vi "capacitance navigation v2.vi"() -> ()   [LabVIEW 2021]
uses:
  <userlib>/Nanonis Prog Interface V5/Nanonis Prog Interface.lvlib
panel:
  out "Delta reached?":bool
  out "Cap reached?":bool
  in  "Cap threshold (pA)":dbl=500.0
  in  "Stop when \nthreshold reached":bool=TRUE
  in  "Stop when delta \nthreshold reached":bool=TRUE
  in  "Delta cap threshold (pA)":dbl=1.0
  in  "pause":bool
  in  "Delete First Entry":bool
  in  "Time between averages (ms)":u32
  out "Avg index":i32
  in  "Averages":i32=50
  in  "milliseconds to wait":u32=1000
  in  "stop":bool
  in  "?":bool
  in  "Max Steps":u16=500
  in  "Direction":enum16{"X +", "X -", "Y +", "Y -", "Z +", "Z -"}(ring)
  out "Delta":cluster{"index":i32, sgl}[](graph)
  in  "Number of Steps":u16=50
  out "Capacitance":cluster{"index":i32, sgl}[](graph)
  in  "Frequency (Hz)":sgl=261.0
  in  "Amplitude (V)":sgl=260.0
  # "Max Steps On"
  # "Max Steps Off"
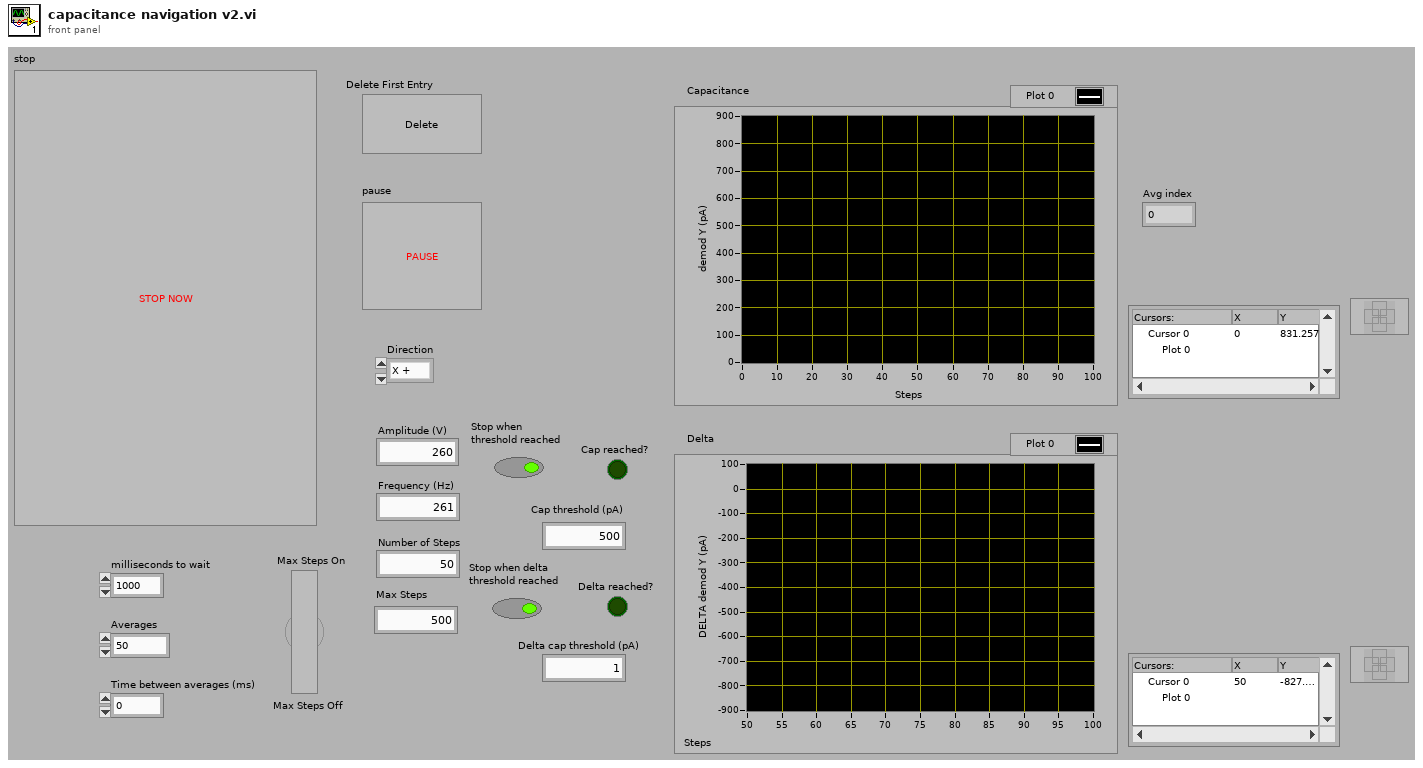
[diagram p1: front panel]
types:
  T1 = enum8{"Group 1", "Group 2", "Group 3", "Group 4", "Group 5", "Group 6"}
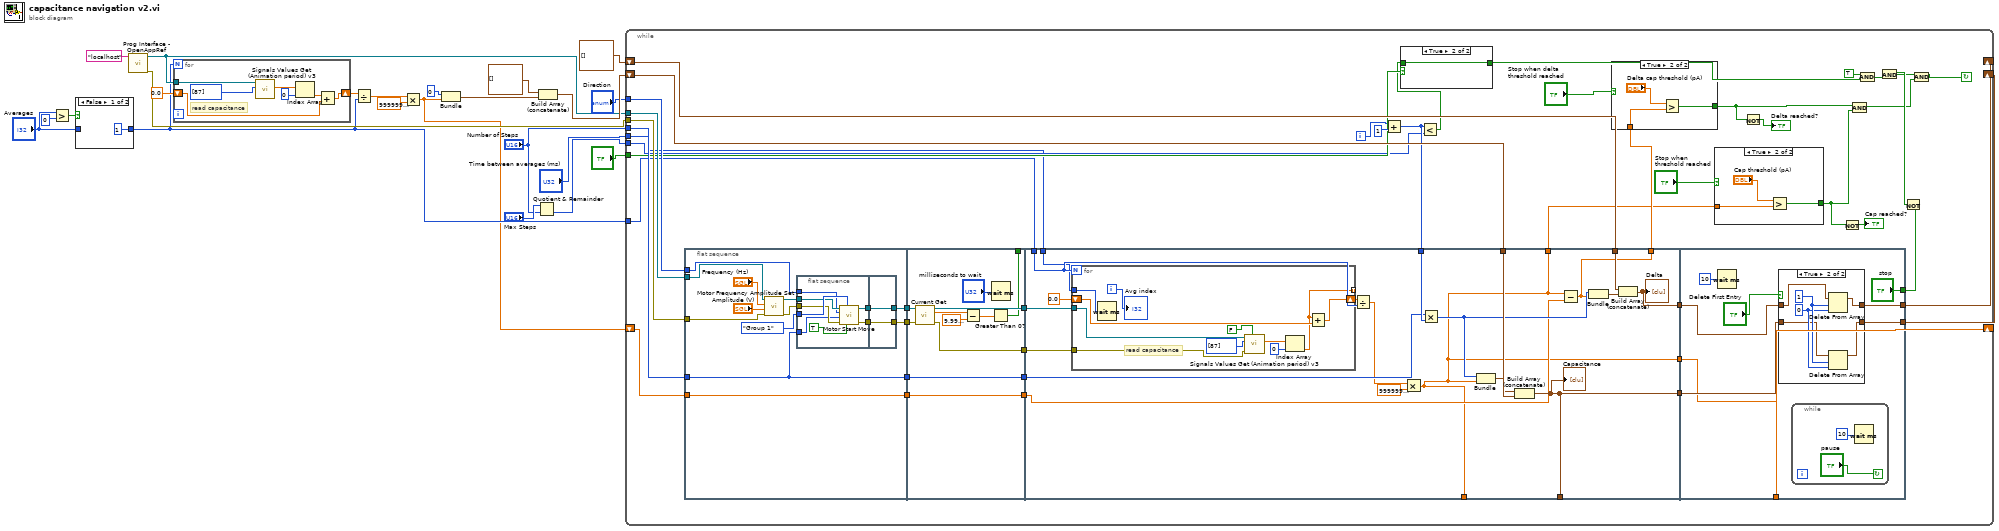
[diagram p0: block diagram]
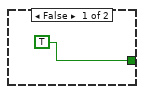
[diagram p3: hidden frame]
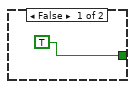
[diagram p4: hidden frame]
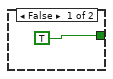
[diagram p5: hidden frame]
diagram:
  n1 = Greater?(x="Averages", y=0) -> (0:w8:bool)
  n2 = case shown="False" w8 {
    tunnel: "Averages" -> [_ w25]
    tunnel: [1 ("Averages") w25] -> w3
    frame False {
    }
    frame True {
    }
  }
  n3 = call <userlib>:"Prog Interface - OpenAppRef.vi"("Machine name (local machine IP)"="localhost" ("machine name (localhost)")) -> ("Error out"=w17:errorcluster, "Application reference"=w16:refnum<vi>)  [unwired: 5 in]
  n4 = for {
    N: w3 -> [_]
    tunnel: w16 -> [w29]
    shift-right: [w26] -> w4
    shift-left: sgl 0.0 ("Internal Ch Value") -> [w28]
    # "read capacitance"
    n5 = call <userlib>:"Signals Values Get (Animation period) v3.vi"("Signals indexes (0-127)"=i8[] [87], "Application ref in"=w29) -> ("Signals Values"=w30:sgl[])  [unwired: 6 in, 2 out]
    n6 = Index Array(array=w30, index=0) -> (element=w27:sgl)
    n7 = Add(x=w27, y=w28) -> (x+y=w26:sgl)
  }
  n8 = Divide(x=w4, y=w3) -> (x/y=w2:sgl)
  n9 = Multiply(x=w2, y=sgl 1000000000000.0) -> (x*y=w1:sgl)
  n10 = Bundle("index"=0, w1) -> (w20:cluster{"index":i32, sgl})  [unwired: 1 in]
  n11 = Quotient & Remainder(x="Max Steps", y="Number of Steps") -> (floor(x/y)=w11:u16)  [unwired: 1 out]
  n12 = Build Array (concatenate)(cluster{i32, sgl}[] [], w20) -> (w19:cluster{"index":i32, sgl}[])
  n13 = while {
    shift-right: [w48] -> _
    shift-left: w19 -> [w75]
    tunnel: w16 -> [w73]
    tunnel: w17 -> [w72]
    shift-right: [w66] -> _
    shift-left: cluster{i32, sgl}[] [] -> [w65]
    tunnel: "Direction" -> [w64]
    tunnel: "Number of Steps" -> [w63]
    tunnel: w11 -> [w56]
    tunnel: "?" -> [w62]
    tunnel: w3 -> [w51]
    tunnel: "Time between averages (ms)" -> [w50]
    shift-right: [w46] -> _
    shift-left: w1 -> [w45]
    i -> [w59]
    stop <- w41 continue-if-true
    n14 = flat-sequence {
      tunnel: [w90] -> w77
      tunnel: w73 -> [w93]
      tunnel: w72 -> [w96]
      tunnel: [w95] -> w71
      tunnel: [w94] -> w70
      tunnel: w64 -> [w89]
      tunnel: w63 -> [w90]
      tunnel: w45 -> [w88]
      tunnel: [w88] -> w44
      tunnel: w77 -> [w122]
      tunnel: [w122] -> w76
      tunnel: w71 -> [w121]
      tunnel: w70 -> [w120]
      tunnel: [w119] -> w69
      tunnel: [w118] -> w68
      tunnel: [w115] -> _
      tunnel: w44 -> [w112]
      tunnel: [w112] -> w43
      tunnel: [w126] -> _
      tunnel: w57 -> [w141]
      tunnel: w76 -> [w138]
      tunnel: w75 -> [w139]
      tunnel: [w123] -> _
      tunnel: w69 -> [w137]
      tunnel: w68 -> [w136]
      tunnel: [w132] -> w67
      tunnel: w65 -> [w133]
      tunnel: w51 -> [w128]
      tunnel: w50 -> [w127]
      tunnel: [w126] -> w49
      tunnel: [w123] -> w47
      tunnel: w43 -> [w125]
      tunnel: [w124] -> w42
      tunnel: [w123] -> w38
      tunnel: w67 -> [w159]
      tunnel: [w158] -> w66
      tunnel: ["stop"] -> w52
      tunnel: [w156] -> w48
      tunnel: w49 -> [w157]
      tunnel: w47 -> [w155]
      tunnel: [w155] -> w46
      frame #0 {
        n15 = call <userlib>:"Motor Frequency Amplitude Set.vi"("Error in (no error)"=w96, "Amplitude (V) (NaN=no change)"="Amplitude (V)", "Frequency (Hz) (NaN=no change)"="Frequency (Hz)", "Application ref in"=w93) -> ("Error out"=w97:errorcluster, "Application ref out"=w98:refnum<vi>)  [unwired: 6 in]
        n16 = flat-sequence {
          tunnel: T1."Group 1" ("Group") -> [w108]
          tunnel: w98 -> [w107]
          tunnel: w97 -> [w106]
          tunnel: w90 -> [w105]
          tunnel: [w104] -> w92
          tunnel: [w103] -> w91
          tunnel: w89 -> [w102]
          tunnel: [w110] -> w94
          tunnel: [w111] -> w95
          tunnel: w92 -> [w111]
          tunnel: w91 -> [w110]
          frame #0 {
            n17 = call <userlib>:"Motor Start Move.vi"("Wait until finished? (F)"=TRUE, "Group"=w108, "Error in (no error)"=w106, "Number of steps"=w105, "Direction"=w102, "Application ref in"=w107) -> ("Error out"=w103:errorcluster, "Application ref out"=w104:refnum<vi>)  [unwired: 3 in]
          }
          frame #1 {
          }
        }
      }
      frame #1 {
        n18 = call <userlib>:"Current Get.vi"("Error in (no error)"=w120, "Application ref in"=w121) -> ("Error out"=w119:errorcluster, "Current (A)"=w117:sgl, "Application ref out"=w118:refnum<vi>)  [unwired: 5 in]
        n19 = Subtract(x=w117, y=sgl 1e-09) -> (x-y=w116:sgl)
        n20 = Greater Than 0?(x=w116) -> (x > 0?=w115:bool)
        n21 = Wait (ms)(milliseconds to wait="milliseconds to wait") -> ()  [unwired: 1 out]
      }
      frame #2 {
        n22 = for {
          N: w128 -> [_]
          tunnel: w137 -> [w150]
          tunnel: w136 -> [w149]
          shift-right: [w147] -> w130
          shift-left: sgl 0.0 ("y") -> [w148]
          tunnel: w127 -> [w145]
          tunnel: [w143] -> _ mode=indexing
          i -> [w146]
          # "read capacitance"
          n23 = Wait (ms)(milliseconds to wait=w145) -> ()  [unwired: 1 out]
          n24 = call <userlib>:"Signals Values Get (Animation period) v3.vi"("Wait for newest data (F=False)"=FALSE, "error in (no error)"=w150, "Signals indexes (0-127)"=i8[] [87], "Application ref in"=w149) -> ("Signals Values"=w151:sgl[])  [unwired: 4 in, 2 out]
          n25 = Index Array(array=w151, index=0) -> (element=w143:sgl)
          n26 = Add(x=w143, y=w148) -> (x+y=w147:sgl)
          "Avg index" <- w146
        }
        n27 = Divide(x=w130, y=w128) -> (x/y=w129:sgl)
        n28 = Multiply(x=w129, y=sgl 1000000000000.0) -> (x*y=w123:sgl)
        n29 = Multiply(x=w138, y=w141) -> (x*y=w135:i32)
        n30 = Bundle(w135, w123) -> (w140:cluster{i32, sgl})  [unwired: 1 in]
        n31 = Build Array (concatenate)(w139, w140) -> (w126:cluster{"index":i32, sgl}[])
        "Capacitance" <- w126
        n32 = Subtract(x=w123, y=w125) -> (x-y=w124:sgl)
        n33 = Bundle(w135, w124) -> (w134:cluster{i32, sgl})  [unwired: 1 in]
        n34 = Build Array (concatenate)(w133, w134) -> (w132:cluster{i32, sgl}[])
        "Delta" <- w132
      }
      frame #3 {
        n35 = Wait (ms)(milliseconds to wait=u32 10) -> ()  [unwired: 1 out]
        n36 = case shown="True" "Delete First Entry" {
          tunnel: w159 -> [w165 w169]
          tunnel: [w165 w168] -> w158
          tunnel: w157 -> [w164 w166]
          tunnel: [w164 w167] -> w156
          frame False {
          }
          frame True {
            w171 = 1 ("length")
            w170 = 0 ("index")
            n37 = Delete From Array(array=w169, length=w171, index=w170) -> (array with subset deleted=w168:cluster{i32, sgl}[])  [unwired: 1 out]
            n38 = Delete From Array(array=w166, length=w171, index=w170) -> (array with subset deleted=w167:cluster{"index":i32, sgl}[])  [unwired: 1 out]
          }
        }
        n39 = while {
          stop <- "pause" continue-if-true
          n40 = Wait (ms)(milliseconds to wait=u32 10) -> ()  [unwired: 1 out]
        }
      }
    }
    n41 = Add(x=w59, y=u16 1) -> (x+y=w57:i32)
    n42 = Less?(x=w57, y=w56) -> (x < y?=w58:bool)
    n43 = case shown="True" w62 {
      tunnel: w58 -> [_ w87]
      tunnel: [TRUE w87] -> w60
      frame False {
      }
      frame True {
      }
    }
    n44 = case shown="True" "Stop when delta \nthreshold reached" {
      tunnel: w42 -> [_ w85]
      tunnel: [TRUE w83] -> w36
      frame False {
      }
      frame True {
        n45 = Greater?(x="Delta cap threshold (pA)", y=w85) -> (0:w83:bool)
      }
    }
    n46 = case shown="True" "Stop when \nthreshold reached" {
      tunnel: w38 -> [_ w80]
      tunnel: [TRUE w79] -> w34
      frame False {
      }
      frame True {
        n47 = Greater?(x="Cap threshold (pA)", y=w80) -> (0:w79:bool)
      }
    }
    n48 = Not(x=w36) -> (.not. x?=→"Delta reached?":bool)
    n49 = Not(x=w34) -> (.not. x?=→"Cap reached?":bool)
    n50 = And(x=w36, y=w34) -> (x .and. y?=w37:bool)
    n51 = And(x=TRUE, y=w60) -> (x .and. y?=w54:bool)
    n52 = Not(x=w52) -> (.not. x?=w55:bool)
    n53 = And(x=w55, y=w54) -> (x .and. y?=w53:bool)
    n54 = And(x=w53, y=w37) -> (x .and. y?=w41:bool)
  }
